vi "GUI TDMS Update.vi"(8 "error in (no error)":errorcluster, 10 "GUI Refs":T1, 11 "View Model":T2) -> (0 "error out":errorcluster, 3 "View Model":T2)   [LabVIEW 2017]
doc: "Update GUI TDMS Cluster by Reference from DVR"
uses:
  View Model/Controls/View Model.ctl
  View Model/Controls/Shared Model.ctl
  Error Handler/Controls/Error Model.ctl
  Error Handler/Controls/Error Event.ctl
  Error Handler/Controls/Error Type.ctl
  Controller/Controls/Controller Model.ctl
  Controller/Controls/Controller Event.ctl
  Controller/Controls/Controller Command.ctl
  Controller/Controls/Controller Overhead.ctl
  Real-Time/RT Status.ctl
  Real-Time/RT Loop Status.ctl
  Controller/Controls/Controller NStream.ctl
  Controller/Controls/Controller Timer Data.ctl
  Controller/Controls/Controller DAQ Data.ctl
  TDMS Logger/Controls/TDMS Model.ctl
  TDMS Logger/Controls/TDMS Event.ctl
  TDMS Logger/Controls/TDMS Command.ctl
  TDMS Logger/Controls/TDMS Overhead.ctl
  TDMS Logger/Controls/TDMS ChanProperties.ctl
  TDMS Logger/Controls/TDMS DAQ Data.ctl
  Controls/GUI Referencies.ctl
  Controls/TDMS_GUI_Cluster.ctl
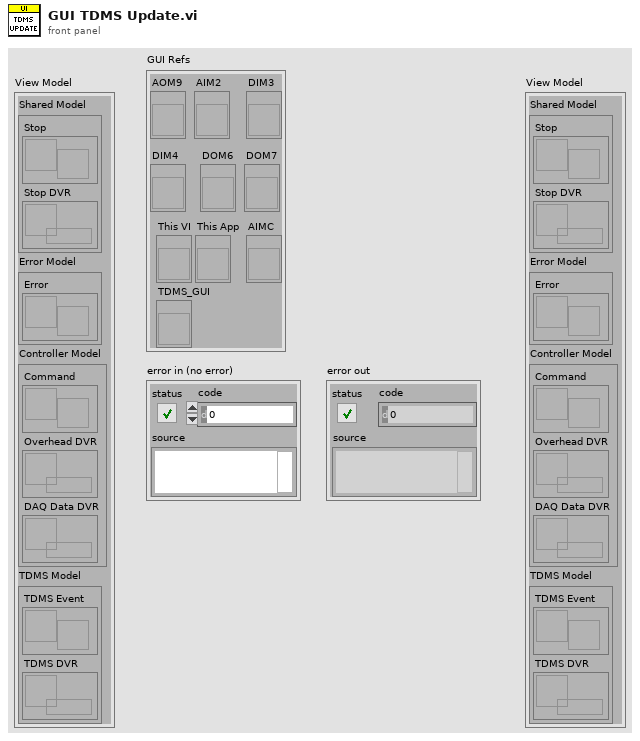
[diagram p1: front panel]
types:
  T1 = typedef "GUI Referencies.ctl" = cluster{"This VI":refnum<vi>, "This App":refnum<vi>, "DIM3":refnum<vi>, "DIM4":refnum<vi>, "DOM6":refnum<vi>, "DOM7":refnum<vi>, "AOM9":refnum<vi>, "AIM2":refnum<vi>, "AIMC":refnum<vi>, "TDMS_GUI":refnum<vi>}
  T2 = typedef "View Model.ctl" = cluster{"Shared Model":T3, "Error Model":T4, "Controller Model":T5, "TDMS Model":T6}
  T3 = typedef "Shared Model.ctl" = cluster{"Stop":refnum<user-event>, "Stop DVR":refnum<data-value>}
  T4 = typedef "Error Model.ctl" = cluster{"Error":refnum<user-event>}
  T5 = typedef "Controller Model.ctl" = cluster{"Command":refnum<user-event>, "Overhead DVR":refnum<data-value>, "DAQ Data DVR":refnum<data-value>}
  T6 = typedef "TDMS Model.ctl" = cluster{"TDMS Event":refnum<user-event>, "TDMS DVR":refnum<data-value>}
  T7 = typedef "TDMS_GUI_Cluster.ctl" = cluster{"FileSize":i32, "FileName":string, "Active?":bool}
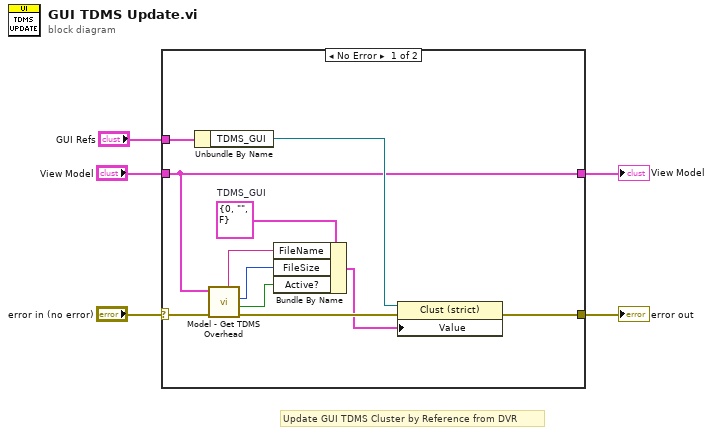
[diagram p0: block diagram]
diagram:
  # "Update GUI TDMS Cluster by Reference from DVR"
  n1 = case shown="No Error" "error in (no error)" {
    selector: "error in (no error)" -> [w13 w17]
    tunnel: [w7 w17] -> w4
    tunnel: "View Model" -> [w6 w18]
    tunnel: [w6 w18] -> w2
    tunnel: "GUI Refs" -> [w16 _]
    frame No Error {
      w14 = T7 {"FileSize"=0, "FileName"="", "Active?"=FALSE}  # TDMS_GUI
      n2 = Unbundle By Name(w16) -> ("TDMS_GUI"=w15:refnum<vi>)
      n3 = call "Model - Get TDMS Overhead.vi"("error in (no error)"=w13, "View Model"=w6) -> ("error out"=w12:errorcluster, "Use TDMS?"=w11:bool, "FileSize"=w9:i32, "FileName"=w10:string)  [unwired: 4 in, 2 out]
      n4 = Bundle By Name(cluster=w14, "FileName"=w10, "FileSize"=w9, "Active?"=w11) -> (w8:T7)
      n5 = property class="Clust (strict)"(reference=w15, error in=w12, "Value"=w8) -> (error out=w7:errorcluster)  [unwired: 1 out]
    }
    frame Error {
    }
  }
  "View Model" <- w2
  "error out" <- w4
